vi "update_filepath.vi"() -> ()   [LabVIEW 2019]
uses:
  <vilib>/Utility/file.llb/Read Delimited Spreadsheet (string).vi
  <vilib>/Utility/file.llb/Write Delimited Spreadsheet (string).vi
panel:
  in  "new_folder":string="C:\\Users\\Administrator\\Documents\\Gillette\\MH6\\YOLO\\darkflow\\train\\Images"
  in  "train_annotations.csv":path=path "C:/Users/Naomi Tan/Documents/Gillette/MH6/videos/Annotations/cropped_data/train_annotations.csv"
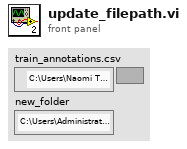
[diagram p1: front panel]
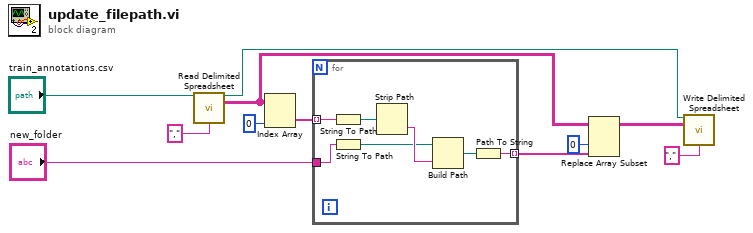
[diagram p0: block diagram]
diagram:
  n1 = call-poly <vilib>:"Read Delimited Spreadsheet.vi"("file path (dialog if empty)"="train_annotations.csv", "delimiter (\\t)"="," ("delimiter (\\t)")) -> ("new file path (Not A Path if cancelled)"=w2:path, "all rows"=w6:string[][])  [unwired: 8 in, 4 out]
  n2 = Index Array(array=w6, index (col)=0 ("disabled index (col)")) -> (element=w8:string[])  [unwired: 1 in]
  n3 = for {
    tunnel: w8 -> [w15] mode=indexing
    tunnel: "new_folder" -> [w14]
    tunnel: [w12] -> w5 mode=indexing
    n4 = String To Path(string=w15) -> (path=w18:path)
    n5 = String To Path(string=w14) -> (path=w16:path)
    n6 = Strip Path(path=w18) -> (name=w17:string)  [unwired: 1 out]
    n7 = Build Path(base path=w16, name or relative path=w17) -> (appended path=w13:path)
    n8 = Path To String(path=w13) -> (string=w12:string)
  }
  n9 = Replace Array Subset(array=w6, new element=w5, index (col)=0 ("disabled index (col)")) -> (w3:string[][])  [unwired: 1 in]
  n10 = call-poly <vilib>:"Write Delimited Spreadsheet.vi"("file path (dialog if empty)"=w2, "2D data"=w3, "delimiter (\\t)"="," ("delimiter (\\t)")) -> ()  [unwired: 11 in, 2 out]
